vi "5 Balls.vi"() -> ()   [LabVIEW 2019]
uses:
  Default5BallEnum.ctl
  Team Code/MotorsGlobal.vi
  Team Code/JoysticksGlobal.vi
panel:
  in  "5BallPID":T1(tab)
  in  "TimeLimit_Anda1":dbl=5000.0
  in  "DistanceAnda1":dbl=-3.2
  in  "DelayAnda1":i32=300
  in  "Anda1Gains":T2={"proportional gain (Kc)"=1.7, "integral time (Ti, min)"=0.008, "derivative time (Td, min)"=0.0} {"derivative time (Td, min)" format="%.3f"; "integral time (Ti, min)" format="%.3f"; "proportional gain (Kc)" format="%.3f"}
  in  "Anda1Range":cluster{"output high":dbl, "output low":dbl}={"output high"=-0.7, "output low"=0.7} {"output low" format="%.2f"; "output high" format="%.2f"}
  in  "Anda2Gains":T2={"proportional gain (Kc)"=1.7, "integral time (Ti, min)"=0.008, "derivative time (Td, min)"=0.0} {"derivative time (Td, min)" format="%.3f"; "integral time (Ti, min)" format="%.3f"; "proportional gain (Kc)" format="%.3f"}
  in  "Anda2Range":cluster{"output high":dbl, "output low":dbl}={"output high"=-0.7, "output low"=0.7} {"output low" format="%.2f"; "output high" format="%.2f"}
  in  "TimeLimit_Anda2":dbl=5000.0
  in  "DistanceAnda2":dbl=-2.9
  in  "Delay After CurvaDir2":i32
  in  "Setpoint_CurvaDir1":dbl=140.0
  in  "GainsCurvaDir1":T2={"proportional gain (Kc)"=1.0, "integral time (Ti, min)"=0.01, "derivative time (Td, min)"=0.0} {"derivative time (Td, min)" format="%.3f"; "integral time (Ti, min)" format="%.3f"; "proportional gain (Kc)" format="%.3f"}
  in  "RangeCurvaDir1":cluster{"output high":dbl, "output low":dbl}={"output high"=0.6, "output low"=-0.6} {"output low" format="%.2f"; "output high" format="%.2f"}
  in  "TimeLimit_CurvaDir1":dbl=5000.0
  in  "Delay After CurvaDir1":i32
  in  "GainsCurvaDir2":T2={"proportional gain (Kc)"=1.0, "integral time (Ti, min)"=0.01, "derivative time (Td, min)"=0.0} {"derivative time (Td, min)" format="%.3f"; "integral time (Ti, min)" format="%.3f"; "proportional gain (Kc)" format="%.3f"}
  in  "RangeCurvaDir2":cluster{"output high":dbl, "output low":dbl}={"output high"=0.6, "output low"=-0.6} {"output low" format="%.2f"; "output high" format="%.2f"}
  in  "Setpoint_CurvaDir2":dbl=40.0
  in  "TimeLimit_CurvaDir1 2":dbl=5000.0
  in  "DelayAnda2":i32=300
  in  "TimeLimit_AlinhaLL":dbl=2000.0
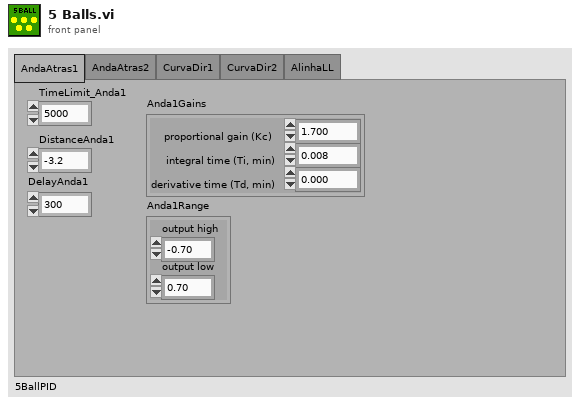
[diagram p1: front panel]
types:
  T1 = enum32{"AndaAtras1", "AndaAtras2", "CurvaDir1", "CurvaDir2", "AlinhaLL"}
  T2 = cluster{"proportional gain (Kc)":dbl, "integral time (Ti, min)":dbl, "derivative time (Td, min)":dbl}
  T3 = typedef "Default5BallEnum.ctl" = enum16{"Reset1", "Anda1", "CurvaDir1", "Reset2", "Anda2", "CurvaDir2", "AlinhaLL", "Atira"}
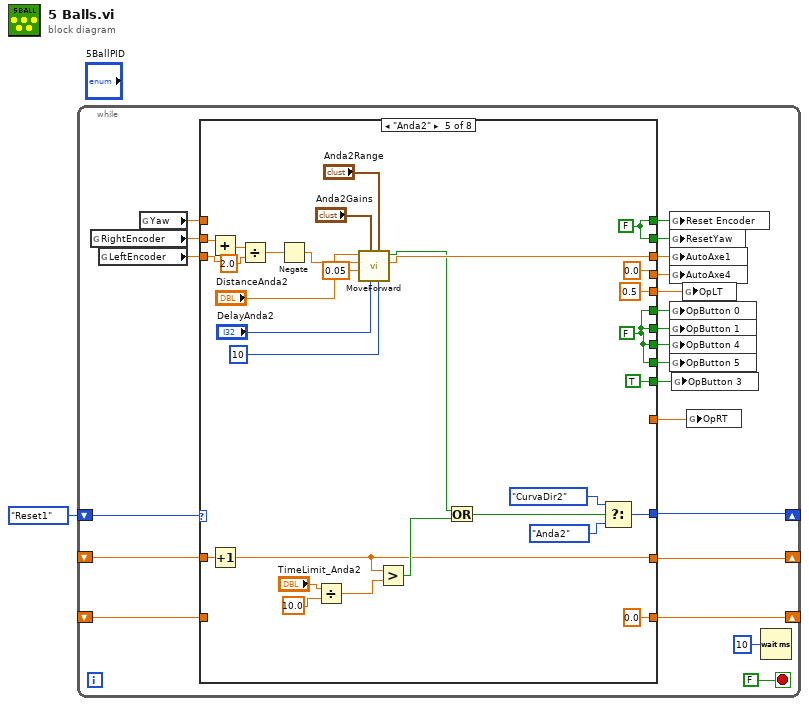
[diagram p0: block diagram]
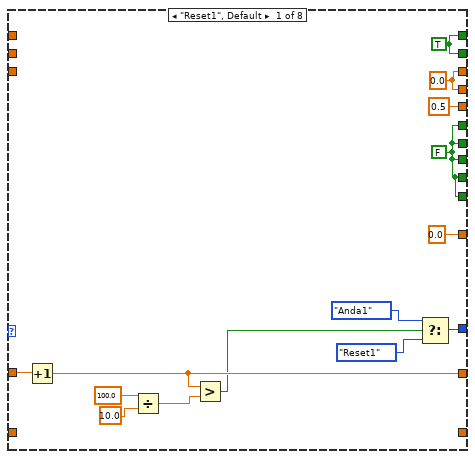
[diagram p2: hidden frame]
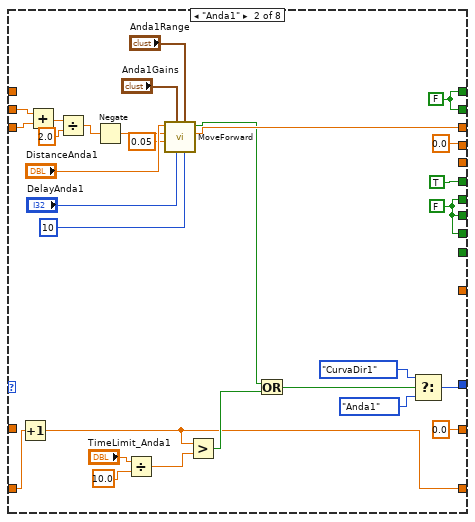
[diagram p3: hidden frame]
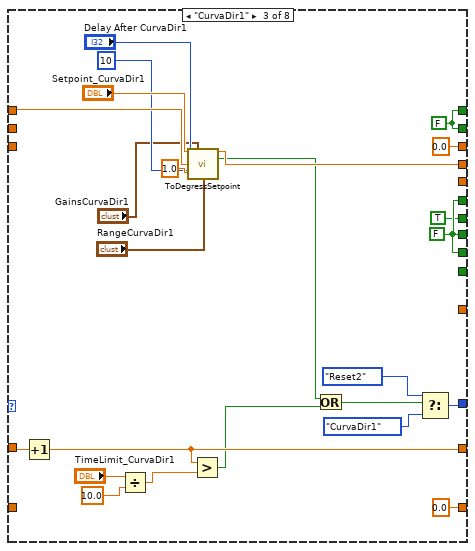
[diagram p4: hidden frame]
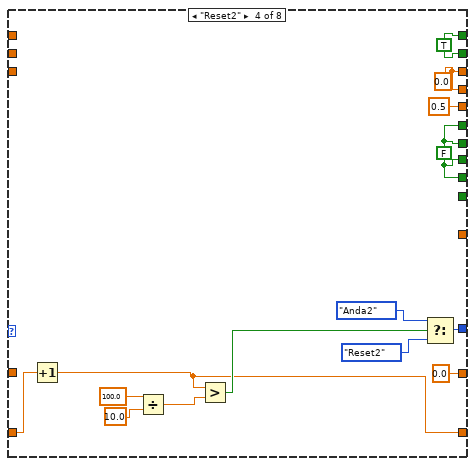
[diagram p5: hidden frame]
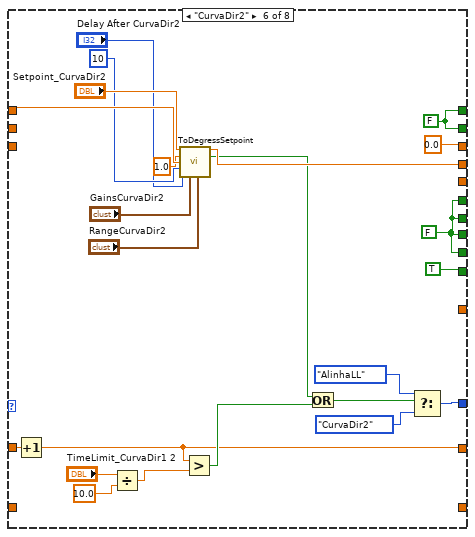
[diagram p6: hidden frame]
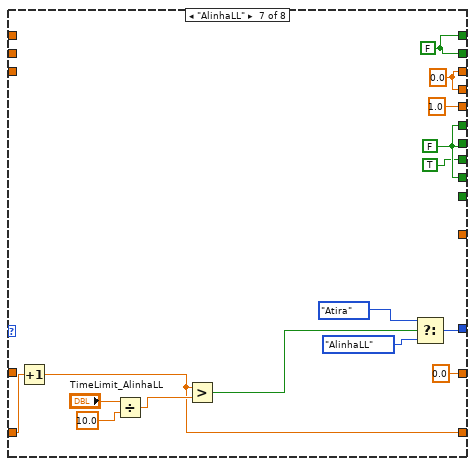
[diagram p7: hidden frame]
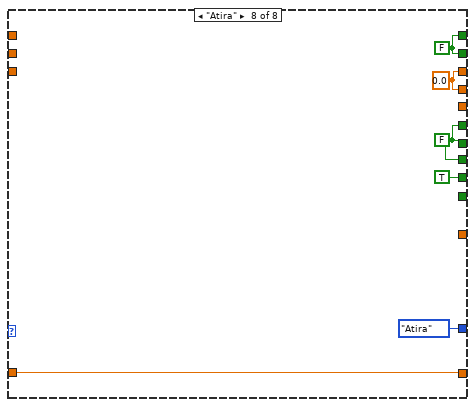
[diagram p8: hidden frame]
diagram:
  n1 = while {
    shift-right: [w20] -> _
    shift-left: Default5BallEnum."Reset1" -> [w21]
    shift-right: [w18] -> _
    shift-left: _ -> [w19]
    shift-right: [w5] -> _
    shift-left: _ -> [w6]
    stop <- FALSE stop-if-true
    n2 = global read "MotorsGlobal.vi" "RightEncoder"() -> (w8:dbl)
    n3 = global read "MotorsGlobal.vi" "LeftEncoder"() -> (w7:dbl)
    n4 = global read "MotorsGlobal.vi" "Yaw"() -> (w9:dbl)
    n5 = case shown="\"Anda2\"" w21 {
      tunnel: [w37 w64 w83 w98 w125 w147 w165 Default5BallEnum."Atira"] -> w20
      tunnel: w19 -> [w33 _ w88 _ w123 w143 _ w173]
      tunnel: [w32 0.0 w84 0.0 w124 w148 0.0 w173] -> w18
      tunnel: [w26 TRUE w82 w97 w126 w145 w172 w177] -> w17
      tunnel: [w26 w59 TRUE w97 w126 w145 w172 w177] -> w16
      tunnel: [w26 w59 w82 w97 w126 w145 TRUE w177] -> w15
      tunnel: [w26 w59 w82 w97 w126 w145 w172 TRUE] -> w14
      tunnel: [w30 w60 w90 w96 w127 w146 w171 w176] -> w13
      tunnel: [w30 w60 w90 w96 w127 w146 w171 w176] -> w12
      tunnel: [w29 w41 0.0 ("Trottle") w95 w110 0.0 ("Trottle") w170 w175] -> w11
      tunnel: [w29 0.0 ("Output") w70 w95 0.0 ("Output") w141 w170 w175] -> w10
      tunnel: w9 -> [_ _ w77 _ _ w149 _ _]
      tunnel: w8 -> [_ w49 _ _ w115 _ _ _]
      tunnel: w7 -> [_ w50 _ _ w116 _ _ _]
      tunnel: w6 -> [_ w55 _ w94 _ _ w161 _]
      tunnel: [_ w54 0.0 w93 0.0 _ w160 _] -> w5
      tunnel: [w26 _ _ _ TRUE TRUE _ _] -> w4
      tunnel: [0.5 _ _ 0.5 0.5 _ 1.0 _] -> w3
      tunnel: [0.0 _ _ _ _ _ _ _] -> w2
      frame "Reset1", Default {
        w29 = 0.0
        w30 = TRUE
        w26 = FALSE
        n6 = Increment(x=w33) -> (x+1=w32:dbl)
        n7 = Divide(x=100.0, y=10.0) -> (x/y=w34:dbl)
        n8 = Greater?(x=w32, y=w34) -> (0:w31:bool)
        n9 = Select(t=Default5BallEnum."Anda1", s=w31, f=Default5BallEnum."Reset1") -> (s? t:f=w37:T3)
      }
      frame "Anda1" {
        w59 = FALSE
        w60 = FALSE
        n10 = Increment(x=w55) -> (x+1=w54:dbl)
        n11 = Add(x=w49, y=w50) -> (x+y=w52:dbl)
        n12 = Divide(x=w52, y=2.0) -> (x/y=w48:dbl)
        n13 = Negate(x=w48) -> (-x=w39:dbl)
        n14 = Divide(x="TimeLimit_Anda1", y=10.0) -> (x/y=w65:dbl)
        n15 = call "MoveForward.vi"("Loop Wait Delay"=10 ("Loop Timer"), "Range"="Anda1Range", "Delay After"="DelayAnda1", "Gains"="Anda1Gains", "Precision"=0.05, "Encoder Count"=w39, "Distance"="DistanceAnda1") -> ("Output"=w41:dbl, "Finished?"=w38:bool)  [unwired: 3 in]
        n16 = Greater?(x=w54, y=w65) -> (0:w61:bool)
        n17 = Or(x=w38, y=w61) -> (x .or. y?=w62:bool)
        n18 = Select(t=Default5BallEnum."CurvaDir1", s=w62, f=Default5BallEnum."Anda1") -> (s? t:f=w64:T3)
      }
      frame "CurvaDir1" {
        w82 = FALSE
        w90 = FALSE
        n19 = Increment(x=w88) -> (x+1=w84:dbl)
        n20 = Divide(x="TimeLimit_CurvaDir1", y=10.0) -> (x/y=w85:dbl)
        n21 = call "ToDegressSetpoint.vi"("Setpoint (degress)"="Setpoint_CurvaDir1", "Gains"="GainsCurvaDir1", "Range"="RangeCurvaDir1", "Yaw"=w77, "Loop Wait Delay"=10, "Delay After"="Delay After CurvaDir1", "Integral Range"=1.0 ("Precision")) -> ("Output"=w70:dbl, "Finished?"=w69:bool)  [unwired: 7 in]
        n22 = Greater?(x=w84, y=w85) -> (0:w75:bool)
        n23 = Or(x=w69, y=w75) -> (x .or. y?=w76:bool)
        n24 = Select(t=Default5BallEnum."Reset2", s=w76, f=Default5BallEnum."CurvaDir1") -> (s? t:f=w83:T3)
      }
      frame "Reset2" {
        w95 = 0.0
        w96 = TRUE
        w97 = FALSE
        n25 = Increment(x=w94) -> (x+1=w93:dbl)
        n26 = Divide(x=100.0, y=10.0) -> (x/y=w102:dbl)
        n27 = Greater?(x=w93, y=w102) -> (0:w101:bool)
        n28 = Select(t=Default5BallEnum."Anda2", s=w101, f=Default5BallEnum."Reset2") -> (s? t:f=w98:T3)
      }
      frame "Anda2" {
        w126 = FALSE
        w127 = FALSE
        n29 = Add(x=w115, y=w116) -> (x+y=w119:dbl)
        n30 = Increment(x=w123) -> (x+1=w124:dbl)
        n31 = Divide(x=w119, y=2.0) -> (x/y=w117:dbl)
        n32 = Negate(x=w117) -> (-x=w114:dbl)
        n33 = Divide(x="TimeLimit_Anda2", y=10.0) -> (x/y=w133:dbl)
        n34 = call "MoveForward.vi"("Loop Wait Delay"=10 ("Loop Timer"), "Range"="Anda2Range", "Delay After"="DelayAnda2", "Gains"="Anda2Gains", "Precision"=0.05, "Encoder Count"=w114, "Distance"="DistanceAnda2") -> ("Output"=w110:dbl, "Finished?"=w107:bool)  [unwired: 3 in]
        n35 = Greater?(x=w124, y=w133) -> (0:w130:bool)
        n36 = Or(x=w107, y=w130) -> (x .or. y?=w131:bool)
        n37 = Select(t=Default5BallEnum."CurvaDir2", s=w131, f=Default5BallEnum."Anda2") -> (s? t:f=w125:T3)
      }
      frame "CurvaDir2" {
        w145 = FALSE
        w146 = FALSE
        n38 = Increment(x=w143) -> (x+1=w148:dbl)
        n39 = Divide(x="TimeLimit_CurvaDir1 2", y=10.0) -> (x/y=w155:dbl)
        n40 = call "ToDegressSetpoint.vi"("Setpoint (degress)"="Setpoint_CurvaDir2", "Gains"="GainsCurvaDir2", "Range"="RangeCurvaDir2", "Precision"=1.0, "Yaw"=w149, "Loop Wait Delay"=10, "Delay After"="Delay After CurvaDir2") -> ("Output"=w141:dbl, "Finished?"=w140:bool)  [unwired: 7 in]
        n41 = Greater?(x=w148, y=w155) -> (0:w152:bool)
        n42 = Or(x=w140, y=w152) -> (x .or. y?=w153:bool)
        n43 = Select(t=Default5BallEnum."AlinhaLL", s=w153, f=Default5BallEnum."CurvaDir2") -> (s? t:f=w147:T3)
      }
      frame "AlinhaLL" {
        w170 = 0.0
        w171 = FALSE
        w172 = FALSE
        n44 = Increment(x=w161) -> (x+1=w160:dbl)
        n45 = Divide(x="TimeLimit_AlinhaLL", y=10.0) -> (x/y=w167:dbl)
        n46 = Greater?(x=w160, y=w167) -> (0:w166:bool)
        n47 = Select(t=Default5BallEnum."Atira", s=w166, f=Default5BallEnum."AlinhaLL") -> (s? t:f=w165:T3)
      }
      frame "Atira" {
        w175 = 0.0
        w176 = FALSE
        w177 = FALSE
      }
    }
    n48 = global write "MotorsGlobal.vi" "Reset Encoder"(w13) -> ()
    n49 = global write "MotorsGlobal.vi" "ResetYaw"(w12) -> ()
    n50 = global write "JoysticksGlobal.vi" "AutoAxe1"(w11) -> ()
    n51 = global write "JoysticksGlobal.vi" "AutoAxe4"(w10) -> ()
    n52 = global write "JoysticksGlobal.vi" "OpButton 0"(w17) -> ()
    n53 = global write "JoysticksGlobal.vi" "OpButton 1"(w16) -> ()
    n54 = global write "JoysticksGlobal.vi" "OpButton 4"(w15) -> ()
    n55 = global write "JoysticksGlobal.vi" "OpButton 5"(w14) -> ()
    n56 = global write "JoysticksGlobal.vi" "OpButton 3"(w4) -> ()
    n57 = global write "JoysticksGlobal.vi" "OpLT"(w3) -> ()
    n58 = global write "JoysticksGlobal.vi" "OpRT"(w2) -> ()
    n59 = Wait (ms)(milliseconds to wait=u32 10) -> ()  [unwired: 1 out]
  }
